vi "vPage_9237x1_CHx1.vi"() -> ()   [LabVIEW 2022 SP3]
uses:
  <vilib>/Utility/sysdir.llb/System Directory Type.ctl
panel:
  out "Buffer":i32
  in  "device name":tag="cDAQ1Mod1"
  in  "¸ê®Æ§¨\nµù°O>":string
  out "DAQ Stoped":bool
  in  "Sample \nto Read":i32=1200
  in  "Sample\nRate":dbl=1200.0
  in  "Enable Saving":bool
  in  "Stop":bool
  out "C1-Save":bool
  out "C1-Trigger":bool
  out "Waveform Chart 2":dynamicdata(graph)
  out "Waveform Chart":dynamicdata(graph)
  # "本頁畫面顯示為 觸發後訊號"
  # "FFT Filter by useing High-pass with Lower Cut-Off (Hz)"
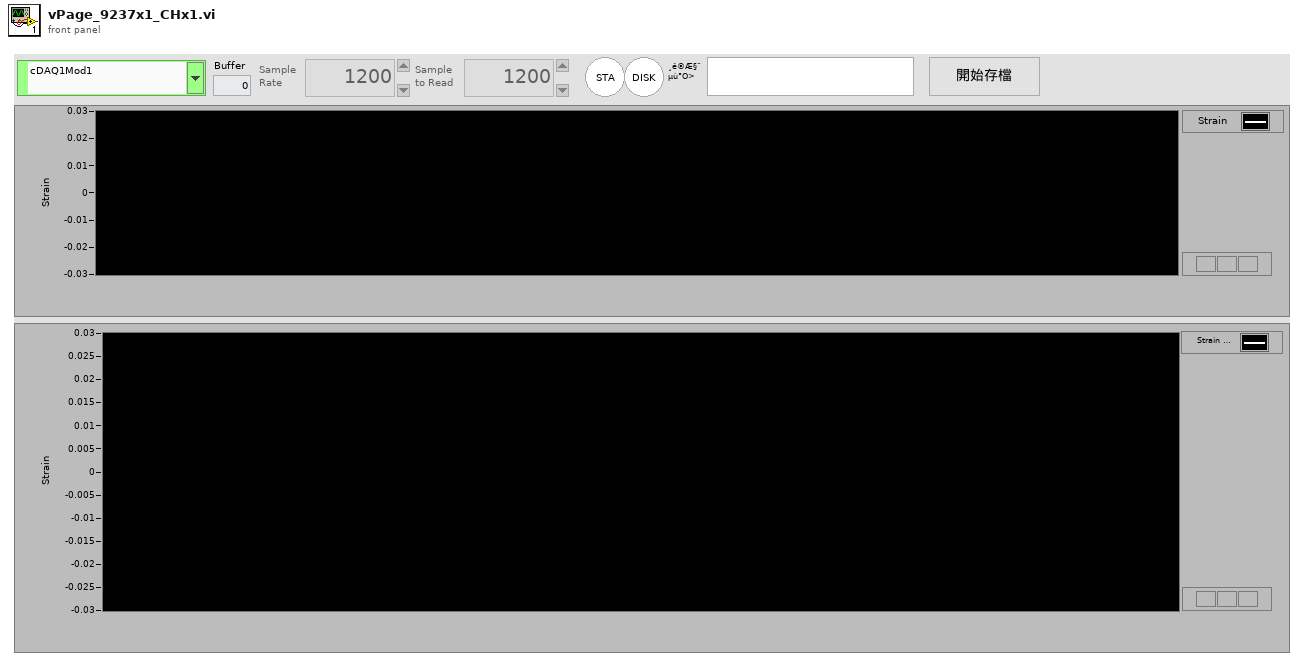
[diagram p1: front panel]
types:
  T1 = enum8{"Enabled", "Disabled", "Disabled and Grayed Out"}
  T2 = typedef "System Directory Type.ctl" = i32
  T3 = cluster{"task out":refnum<k21>, "data":dynamicdata}
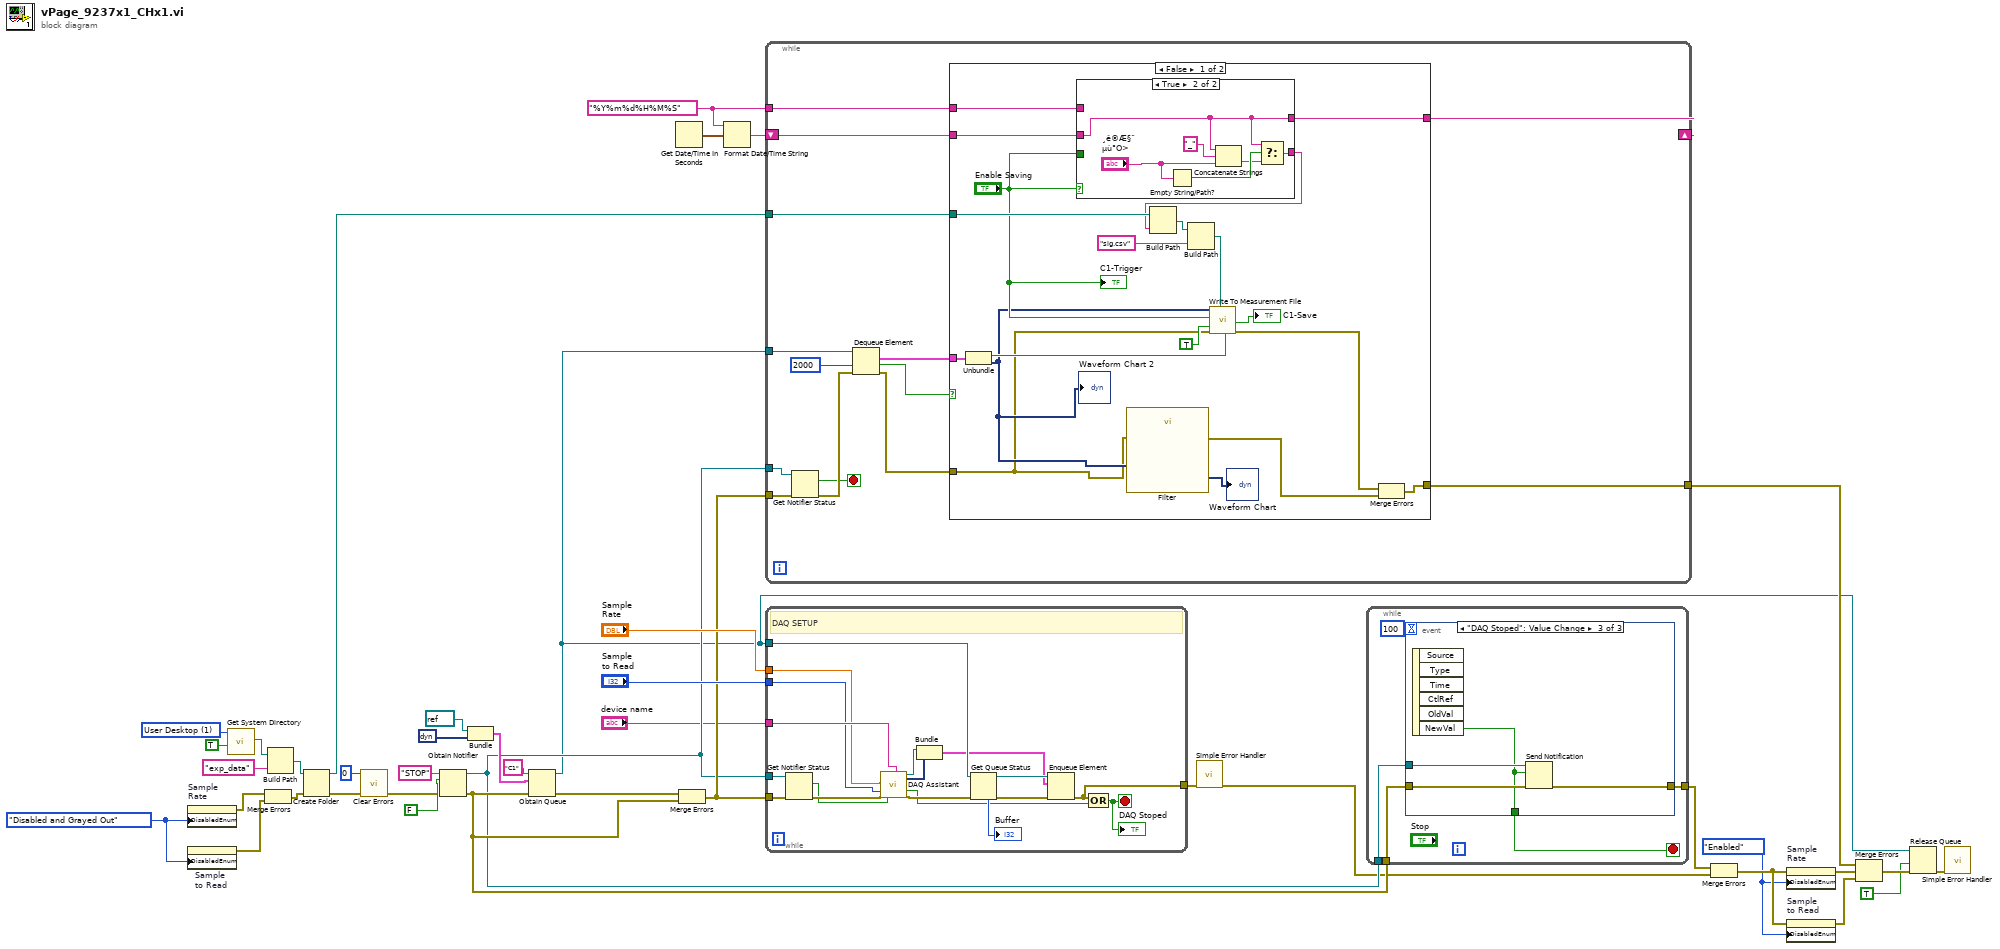
[diagram p0: block diagram]
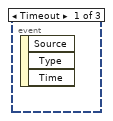
[diagram p2: hidden frame]
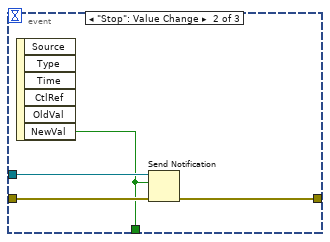
[diagram p3: hidden frame]
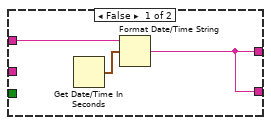
[diagram p4: hidden frame]
diagram:
  w11 = T1."Enabled" ("Disabled")
  w16 = T1."Disabled and Grayed Out" ("Disabled")
  w17 = "%Y%m%d%H%M%S" ("time format string (%c)")
  w26 = T2 1 items=["User Home"=0, "User Desktop"=1, "User Documents"=2, "User Application Data"=3, "User Preferences"=4, "User Temporary"=5, "Public Documents"=6, "Public Application Data"=7, "Public Preferences"=8, "Public Cache"=13, "System Core Libraries"=9, "System Installed Libraries"=10, "Application Files"=11, "Boot Volume Root"=12] ("system directory type")
  n1 = property on="Sample\nRate" class="DigNum (strict)"("DisabledEnum"=w16) -> (error out=w15:errorcluster)  [unwired: 2 in, 1 out]
  n2 = property on="Sample \nto Read" class="DigNum (strict)"("DisabledEnum"=w16) -> (error out=w13:errorcluster)  [unwired: 2 in, 1 out]
  n3 = call <vilib>:"Get System Directory.vi"("create directory if not found? (F)"=TRUE, "system directory type"=w26) -> ("system directory"=w28:path)  [unwired: 9 in]
  n4 = Merge Errors(w15, w13) -> (w14:errorcluster)
  n5 = Build Path(base path=w28, name or relative path="exp_data") -> (appended path=w22:path)
  n6 = Create Folder(path (use dialog)=w22, error in=w14) -> (created path=w21:path, error out=w24:errorcluster)  [unwired: 1 in, 1 out]
  n7 = call <vilib>:"Clear Errors.vi"("error in (no error)"=w24, "specific error code to clear (0: all)"=0) -> ("error out"=w23:errorcluster)  [unwired: 4 in, 1 out]
  n8 = Obtain Notifier(name (unnamed)="STOP", notification data type=FALSE, error in (no error)=w23) -> (notifier out=w18:refnum<notifier>, error out=w20:errorcluster)  [unwired: 1 in, 1 out]
  n9 = Bundle("task out"=refnum<k21> refnum, "data"=dynamicdata []) -> (w33:T3)  [unwired: 1 in]
  n10 = Obtain Queue(name (unnamed)="C1", element data type=w33, error in (no error)=w20) -> (queue out=w5:refnum<queue>, error out=w41:errorcluster)  [unwired: 2 in, 1 out]
  n11 = Get Date/Time In Seconds() -> (seconds since 1Jan1904=w31:timestamp)
  n12 = Merge Errors(w41, w20) -> (w32:errorcluster)
  n13 = Format Date/Time String(time format string (%c)=w17, seconds (now)=w31) -> (date/time string=w30:string)  [unwired: 1 in]
  n14 = while {
    tunnel: w32 -> [w55]
    tunnel: w18 -> [w53]
    tunnel: w5 -> [w52]
    shift-right: [w42] -> _
    shift-left: w30 -> [w46]
    tunnel: w21 -> [w47]
    tunnel: [w43] -> w6
    tunnel: w17 -> [w45]
    stop <- w50 stop-if-true
    n15 = Get Notifier Status(notifier=w53, error in (no error)=w55) -> (current notification=w50:bool, error out=w54:errorcluster)  [unwired: 3 out]
    n16 = Dequeue Element(queue=w52, timeout in ms (-1)=2000, error in (no error)=w54) -> (element=w48:T3, timed out?=w49:bool, error out=w44:errorcluster)  [unwired: 1 out]
    n17 = case shown="False" w49 {
      tunnel: w48 -> [w74 _]
      tunnel: w44 -> [w58 w84]
      tunnel: w46 -> [w72 w85]
      tunnel: [w71 w85] -> w42
      tunnel: w47 -> [w70 _]
      tunnel: [w65 w84] -> w43
      tunnel: w45 -> [w63 _]
      frame False {
        n18 = Unbundle(w74) -> ("task out"=w73:refnum<k21>, "data"=w59:dynamicdata)
        "Waveform Chart 2" <- w59
        n19 = case shown="True" "Enable Saving" {
          tunnel: [w75 w79] -> w71
          tunnel: "Enable Saving" -> [_ _]
          tunnel: w72 -> [_ w79]
          tunnel: [w75 w81] -> w64
          tunnel: w63 -> [w76 _]
          frame False {
            n20 = Get Date/Time In Seconds() -> (seconds since 1Jan1904=w77:timestamp)
            n21 = Format Date/Time String(time format string (%c)=w76, seconds (now)=w77) -> (date/time string=w75:string)  [unwired: 1 in]
          }
          frame True {
            n22 = Empty String/Path?(string/path="¸ê®Æ§¨\nµù°O>") -> (empty?=w83:bool)
            n23 = Concatenate Strings(w79, "_" ("string"), "¸ê®Æ§¨\nµù°O>") -> (w82:string)
            n24 = Select(t=w79, s=w83, f=w82) -> (s? t:f=w81:string)
          }
        }
        n25 = call "Filter"("error in (no error)"=w58, "Signal"=w59) -> ("error out"=w57:errorcluster, "Filtered Signal"=→"Waveform Chart":dynamicdata)  [unwired: 8 in]
        n26 = Build Path(base path=w70, name or relative path=w64) -> (appended path=w69:path)
        n27 = Build Path(base path=w69, name or relative path="sig.csv") -> (appended path=w67:path)
        n28 = call "Write To Measurement File"("Signals"=w59, "Enable"="Enable Saving", "new_file"=TRUE, "error in (no error)"=w58, "Filename"=w67, "DAQmx Task"=w73) -> ("Saving Data"=→"C1-Save":bool, "error out"=w66:errorcluster)  [unwired: 11 in, 1 out]
        n29 = Merge Errors(w66, w57) -> (w65:errorcluster)
        "C1-Trigger" <- "Enable Saving"
      }
      frame True {
      }
    }
  }
  n30 = while {
    tunnel: [w102] -> w2
    tunnel: w5 -> [w99]
    tunnel: w32 -> [w98]
    tunnel: w18 -> [w97]
    tunnel: "Sample \nto Read" -> [w88]
    tunnel: "Sample\nRate" -> [w89]
    tunnel: "device name" -> [w90]
    stop <- w100 stop-if-true
    # "DAQ SETUP"
    n31 = Get Notifier Status(notifier=w97, error in (no error)=w98) -> (current notification=w87:bool, error out=w94:errorcluster)  [unwired: 3 out]
    n32 = call "DAQ Assistant"("rate"=w89, "timeout (s)"=w88, "error in"=w94, "stop (F)"=w87, "device name"=w90) -> ("task out"=w92:refnum<k21>, "data"=w91:dynamicdata, "stopped"=w86:bool, "error out"=w93:errorcluster)  [unwired: 11 in]
    n33 = Bundle("task out"=w92, "data"=w91) -> (w95:T3)  [unwired: 1 in]
    n34 = Get Queue Status(queue=w99, error in (no error)=w93) -> (queue out=w96:refnum<queue>, error out=w103:errorcluster, # elements in queue=→"Buffer":i32)  [unwired: 1 in, 5 out]
    n35 = Enqueue Element(queue=w96, element=w95, error in (no error)=w103) -> (error out=w102:errorcluster)  [unwired: 1 in, 2 out]
    n36 = Compound Arithmetic op=OR(w102, w86) -> (w100:bool)
    "DAQ Stoped" <- w100
  }
  n37 = call <vilib>:"Simple Error Handler.vi"("error in (no error)"=w2) -> ("error out"=w1:errorcluster)  [unwired: 4 in, 4 out]
  n38 = while {
    tunnel: w20 -> [w108]
    tunnel: [w107] -> w19
    tunnel: w18 -> [w106]
    stop <- w105 stop-if-true
    n39 = event shown="[2] \"DAQ Stoped\": Value Change" {
      selector: _ -> [_ _ _]
      dyn-events: _ -> [_ _ _]
      timeout: 100 -> [_ _ _]
      tunnel: w108 -> [_ w112 w116]
      tunnel: [_ w111 w115] -> w107
      tunnel: w106 -> [_ w110 w114]
      tunnel: [_ w109 w113] -> w105
      event Timeout {
        n40 = event-data() -> ()  [unwired: 1 in, 3 out]
      }
      event "Stop": Value Change {
        n41 = event-data() -> ("NewVal"=w109:bool)  [unwired: 1 in, 5 out]
        n42 = Send Notification(notification=w109, notifier=w110, error in (no error)=w112) -> (error out=w111:errorcluster)  [unwired: 1 out]
      }
      event "DAQ Stoped": Value Change {
        n43 = event-data() -> ("NewVal"=w113:bool)  [unwired: 1 in, 5 out]
        n44 = Send Notification(notification=w113, notifier=w114, error in (no error)=w116) -> (error out=w115:errorcluster)  [unwired: 1 out]
      }
    }
  }
  n45 = Merge Errors(w19, w1) -> (w12:errorcluster)
  n46 = property on="Sample\nRate" class="DigNum (strict)"(error in=w12, "DisabledEnum"=w11) -> (error out=w10:errorcluster)  [unwired: 1 in, 1 out]
  n47 = property on="Sample \nto Read" class="DigNum (strict)"(error in=w12, "DisabledEnum"=w11) -> (error out=w9:errorcluster)  [unwired: 1 in, 1 out]
  n48 = Merge Errors(w6, w10, w9) -> (w7:errorcluster)
  n49 = Release Queue(queue=w5, force destroy? (F)=TRUE, error in (no error)=w7) -> (error out=w8:errorcluster)  [unwired: 2 out]
  n50 = call <vilib>:"Simple Error Handler.vi"("error in (no error)"=w8) -> ()  [unwired: 4 in, 5 out]
